vi "Remove.vi"(0 "LV MDI in":refnum<class "LV MDI.lvclass">, 5 "Doc Name[]":string[](array[string]), 11 "error in (no error)":errorcluster) -> (4 "LV MDI out":refnum<class "LV MDI.lvclass">, 6 "Doc Name out[]":string[](array[string]), 15 "error out":errorcluster)   [LabVIEW 2016, in "LV MDI.lvclass"]
doc: "Unload Documents from memory"
uses:
  LV MDI.lvclass
  LV MDI.lvclass/LV MDI.ctl
  Document/Document.lvclass/Document.ctl
  Document/Document.lvclass
  user32.dll
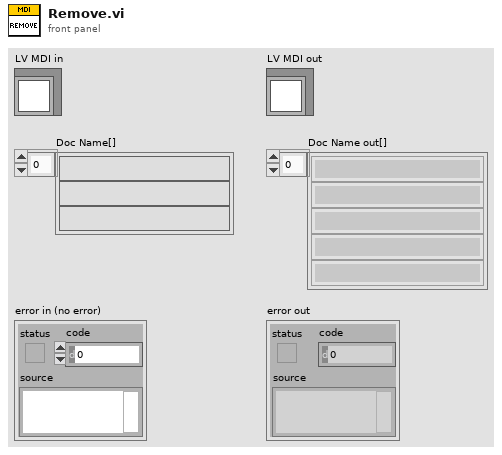
[diagram p1: front panel]
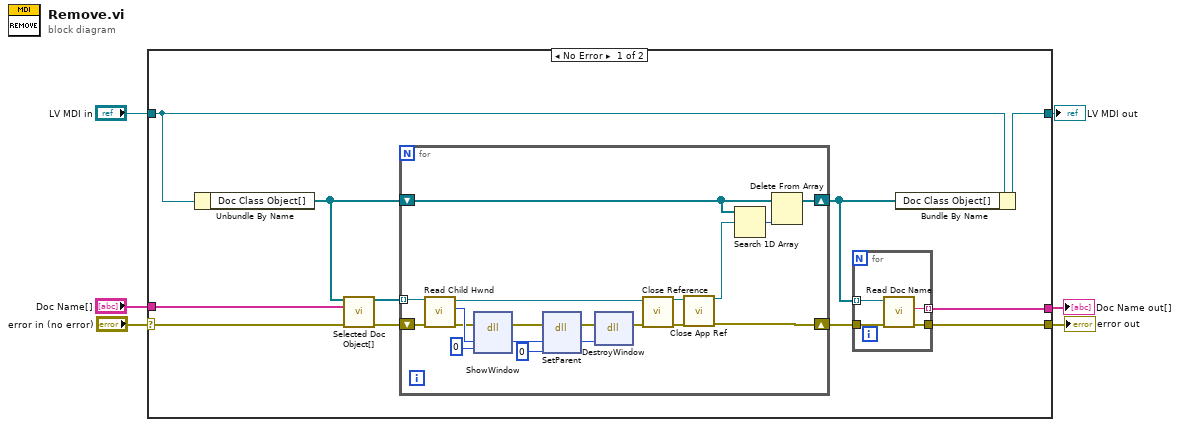
[diagram p0: block diagram]
diagram:
  n1 = case shown="No Error" "error in (no error)" {
    selector: "error in (no error)" -> [w15 w42]
    tunnel: [w9 w42] -> w5
    tunnel: [w17 w41] -> w3
    tunnel: "LV MDI in" -> [w16 w41]
    tunnel: "Doc Name[]" -> [w11 _]
    tunnel: [w7 _] -> w1
    frame No Error {
      n2 = Unbundle By Name(w16) -> ("Doc Class Object[]"=w13:refnum<class "Document.lvclass">[])
      n3 = call "Selected Doc Object[].vi"("Doc Class Object[]"=w13, "Doc Name[]"=w11, "error in"=w15) -> ("Selected Doc[]"=w12:refnum<class "Document.lvclass">[], "error Out"=w14:errorcluster)  [unwired: 11 in]
      n4 = for {
        shift-right: [w24] -> w10
        shift-left: w14 -> [w28]
        tunnel: w12 -> [w29] mode=indexing
        shift-right: [w38] -> w8
        shift-left: w13 -> [w40]
        n5 = call "Read Child Hwnd.vi"("error in (no error)"=w28, "Document in"=w29) -> ("error out"=w31:errorcluster, "Child Hwnd"=w33:u32, "Document out"=w23:refnum<class "Document.lvclass">)  [unwired: 7 in]
        n6 = dll-call lib="user32.dll" fn="ShowWindow"(error in=w31, "hwnd"=w33, "nCmdShow"=u32 0) -> (error out=w30:errorcluster, "hwnd"=w32:u32)  [unwired: 4 in, 1 out]
        n7 = dll-call lib="user32.dll" fn="SetParent"(error in=w30, "Child"=w32, "NewParent"=0) -> (error out=w36:errorcluster, "Child"=w35:u32)  [unwired: 4 in, 1 out]
        n8 = dll-call lib="user32.dll" fn="DestroyWindow"(error in=w36, "hwnd"=w35) -> (error out=w25:errorcluster)  [unwired: 4 in, 1 out]
        n9 = call-dynamic "Close Reference.vi"("Document in"=w23, "error in (no error)"=w25) -> ("Document out"=w26:refnum<class "Document.lvclass">, "error out"=w27:errorcluster)  [unwired: 12 in]
        n10 = call-dynamic "Close App Ref.vi"("Document in"=w26, "error in (no error)"=w27) -> ("Document out"=w22:refnum<class "Document.lvclass">, "error out"=w24:errorcluster)  [unwired: 12 in]
        n11 = Search 1D Array(1D array=w40, element=w22) -> (index of element=w39:i32)  [unwired: 1 in]
        n12 = Delete From Array(array=w40, index=w39) -> (array with subset deleted=w38:refnum<class "Document.lvclass">[])  [unwired: 1 in, 1 out]
      }
      n13 = for {
        tunnel: [w20] -> w9
        tunnel: w10 -> [w21]
        tunnel: w8 -> [w19] mode=indexing
        tunnel: [w18] -> w7 mode=indexing
        n14 = call "Read Doc Name.vi"("error in (no error)"=w21, "Document in"=w19) -> ("error out"=w20:errorcluster, "Doc Name"=w18:string)  [unwired: 7 in, 1 out]
      }
      n15 = Bundle By Name(cluster=w16, "Doc Class Object[]"=w8) -> (w17:refnum<class "LV MDI.lvclass">)
    }
    frame Error {
    }
  }
  "error out" <- w5
  "LV MDI out" <- w3
  "Doc Name out[]" <- w1
